vi "getTestList.vi"(8 "error in (no error)":errorcluster, 10 "listaPruebas":refnum<vi>, 11 "Equipo in":refnum<class "Equipo.lvclass">) -> (0 "error out":errorcluster, 2 "listaDePruebas":refnum<class "Prueba.lvclass">[](array[class]), 3 "Equipo out":refnum<class "Equipo.lvclass">)   [LabVIEW 2019, in "Equipo.lvclass"]
uses:
  Equipo.lvclass
  Pruebas/Prueba/Prueba.lvclass
  Equipo.lvclass/Equipo.ctl
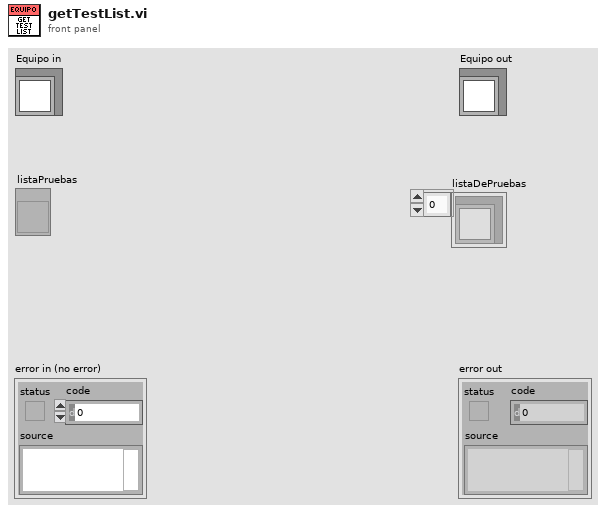
[diagram p1: front panel]
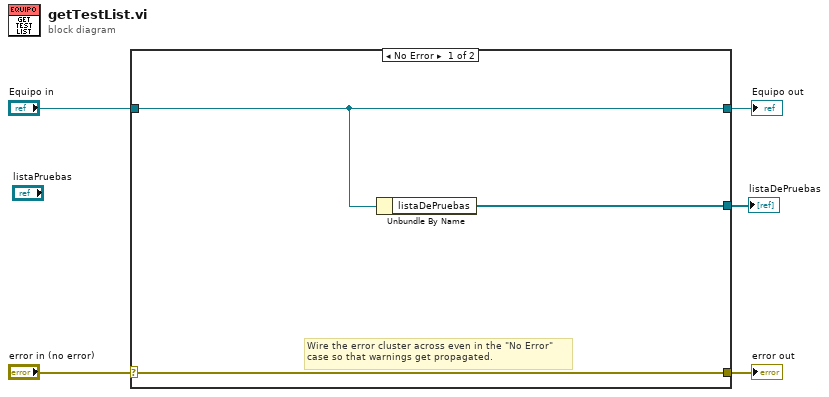
[diagram p0: block diagram]
diagram:
  n1 = case shown="No Error" "error in (no error)" {
    selector: "error in (no error)" -> [w8 w10]
    tunnel: [w8 w10] -> w4
    tunnel: [w7 w9] -> w2
    tunnel: "Equipo in" -> [w7 w9]
    tunnel: [w6 _] -> w1
    frame No Error {
      # "Wire the error cluster across even in the \"No Error\"\ncase so that warnings get propagated."
      n2 = Unbundle By Name(w7) -> ("listaDePruebas"=w6:refnum<class "Prueba.lvclass">[])
    }
    frame Error {
    }
  }
  "error out" <- w4
  "Equipo out" <- w2
  "listaDePruebas" <- w1
